vi "GT Set Enc Response Check.vi"(6 "time":i32, 7 "minEncVel":dbl, 8 "error in (no error)":errorcluster caption="错误输入（无错误）", 9 "dacThreshold":i16, 10 "control":i16, 11 "cardNum":i16) -> (0 "error out":errorcluster caption="错误输出", 3 "function return":i16)   [LabVIEW 2014, in "gts.lvlib"]
doc: "GT_API GT_SetEncResponseCheck(short cardNum,short control,short dacThreshold,double minEncVel,long time);"
uses:
  gts.lvlib
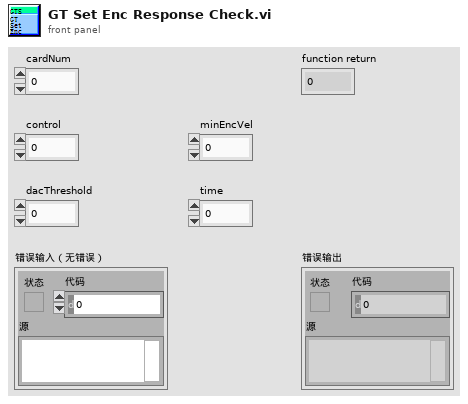
[diagram p1: front panel]
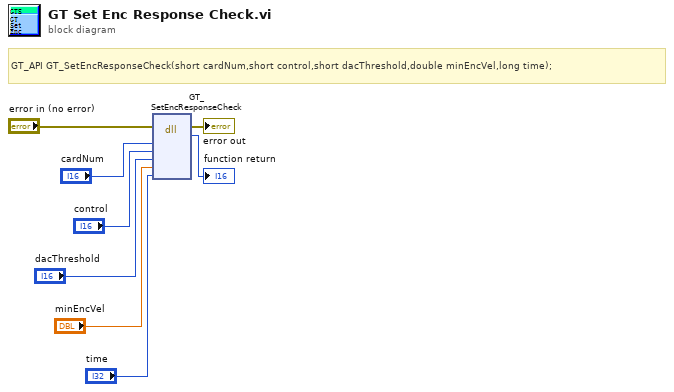
[diagram p0: block diagram]
diagram:
  # "GT_API GT_SetEncResponseCheck(short cardNum,short control,short dacThreshold,double minEncVel,long time);"
  n1 = dll-call lib="PTH2habs D固高科技资料GTS控制卡GTS卡18年上半年资料dllVC32bit\nmulti_cardgts.*" fn="GT_SetEncResponseCheck"(error in="error in (no error)", "cardNum"="cardNum", "control"="control", "dacThreshold"="dacThreshold", "minEncVel"="minEncVel", "time"="time") -> (error out=→"error out":errorcluster, →"function return":i16)  [unwired: 7 in, 1 out]
